vi "FTW-VIServer-VI-Metadata.vi"(0 "VI Filepath":path, 11 "error in":errorcluster) -> (4 "Front Panel Title":string, 6 "VI Description":string, 15 "error out":errorcluster)   [LabVIEW 2013]
panel:
  # "Inputs"
  # "Outputs"
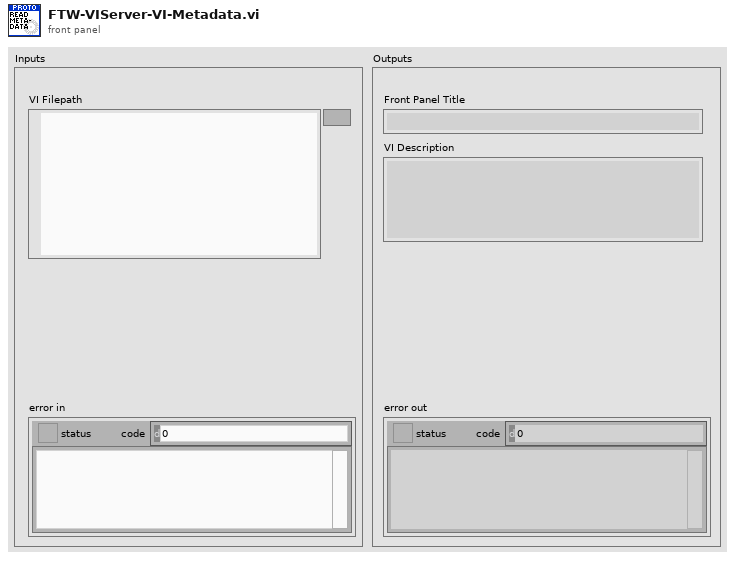
[diagram p1: front panel]
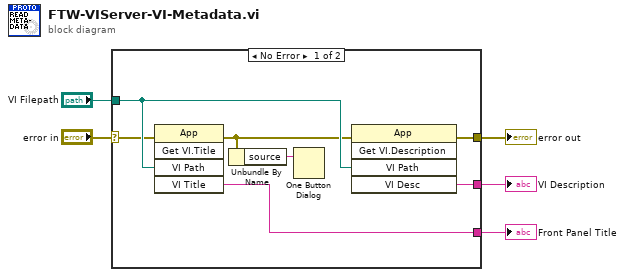
[diagram p0: block diagram]
diagram:
  n1 = case shown="No Error" "error in" {
    selector: "error in" -> [w9 w13]
    tunnel: [w8 w13] -> w5
    tunnel: [w11 _] -> w3
    tunnel: [w10 _] -> w2
    tunnel: "VI Filepath" -> [w12 _]
    frame No Error {
      n2 = invoke class="App" method="Get VI.Title"(error in=w9, "VI Path"=w12) -> (error out=w7:errorcluster, "VI Title"=w11:string)  [unwired: 3 in, 3 out]
      n3 = Unbundle By Name(w7) -> ("source"=w6:string)
      n4 = One Button Dialog(message=w6) -> ()  [unwired: 1 in, 1 out]
      n5 = invoke class="App" method="Get VI.Description"(error in=w7, "VI Path"=w12) -> (error out=w8:errorcluster, "VI Desc"=w10:string)  [unwired: 3 in, 3 out]
    }
    frame Error {
    }
  }
  "error out" <- w5
  "Front Panel Title" <- w3
  "VI Description" <- w2
